vi "Configure Timebase.vi"(7 "Record Length (10000)":u32=10000 caption="Record Length (10000s)", 8 "error in (no error)":errorcluster, 9 "Position (0.0 s)":dbl=50.0, 10 "Timebase (4 ns)":dbl=4.0, 11 "VISA resource name":refnum<visa-resource-name>) -> (0 "error out":errorcluster, 3 "VISA resource name out":refnum<visa-resource-name>)   [LabVIEW 2015, in "Tektronix 7000 Series.lvlib"]
doc: "Configures the timebase and horizontal properties of an oscilloscope."
uses:
  <instrlib>/Tektronix 7000 Series/Tektronix 7000 Series.lvlib
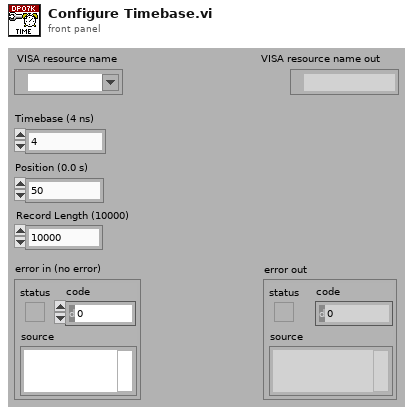
[diagram p1: front panel]
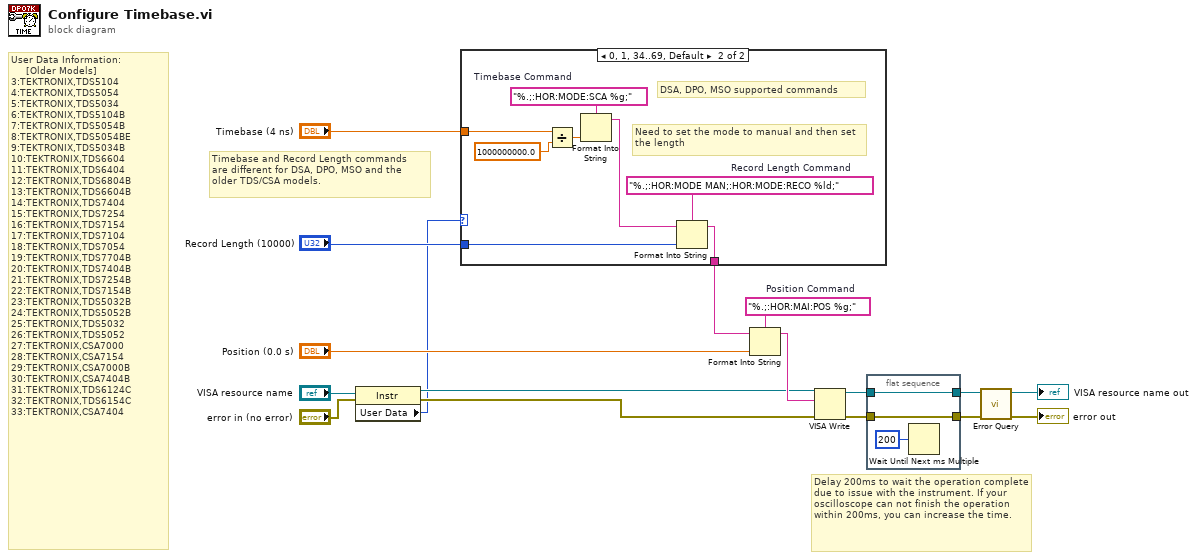
[diagram p0: block diagram]
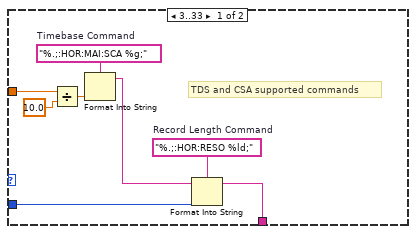
[diagram p2: hidden frame]
diagram:
  w17 = "%.;:HOR:MAI:POS %g;"  # Position Command
  # "Timebase and Record Length commands\nare different for DSA, DPO, MSO and the \nolder TDS/CSA models."
  # "User Data Information:\n     [Older Models]\n3:TEKTRONIX,TDS5104\n4:TEKTRONIX,TDS5054\n5:TEKTRONIX,TDS5034\n6:TEKTRONIX,TDS5104B\n7:TEKTRONIX,TDS5054B\n8:TEKTRONIX,TDS5054BE\n9:TEKTRONIX,TDS5034B\n10:TEKTRONIX,TDS6604\n11:TEKTRONIX,TDS6404\n12:TEKTRONIX,TDS6804B\n13:TEKTRONIX,TDS6604B\n14:TEKTRONIX,TDS7404\n15:TEKTRONIX,TDS7254\n16:TEKTRONIX,TDS7154\n17:TEKTRONIX,TDS7104\n18:TEKTRONIX,TDS7054\n19:TEKTRONIX,TDS7704B\n20:TEKTRONIX,TDS7404B\n21:TEKTRONIX,TDS7254B\n22:TEKTRONIX,TDS7154B\n23:TEKTRONIX,TDS5032B\n24:TEKTRONIX,TDS5052B\n25:TEKTRONIX,TDS5032\n26:TEKTRONIX,TDS5052\n27:TEKTRONIX,CSA7000\n28:TEKTRONIX,CSA7154\n29:TEKTRONIX,CSA7000B\n30:TEKTRONIX,CSA7404B\n31:TEKTRONIX,TDS6124C\n32:TEKTRONIX,TDS6154C\n33:TEKTRONIX,CSA7404"
  # "Delay 200ms to wait the operation complete due to issue with the instrument. If your oscilloscope can not finish the operation within 200ms, you can increase the time."
  n1 = property class="Instr"(reference="VISA resource name", error in="error in (no error)") -> (reference out=w3:refnum<visa-resource-name>, error out=w2:errorcluster, "User Data"=w1:u32)
  n2 = case shown="0, 1, 34..69, Default" w1 {
    tunnel: "Timebase (4 ns)" -> [w20 w31]
    tunnel: "Record Length (10000)" -> [w19 w28]
    tunnel: [w18 w26] -> w6
    frame 3..33 {
      w24 = "%.;:HOR:RESO %ld;"  # Record Length Command
      w25 = "%.;:HOR:MAI:SCA %g;"  # Timebase Command
      # "TDS and CSA supported commands"
      n3 = Divide(x=w20, y=10.0) -> (x/y=w22:dbl)
      n4 = Format Into String(format string=w25, w22) -> (resulting string=w21:string)  [unwired: 2 in, 1 out]
      n5 = Format Into String(format string=w24, initial string=w21, w19) -> (resulting string=w18:string)  [unwired: 1 in, 1 out]
    }
    frame 0, 1, 34..69, Default {
      w32 = "%.;:HOR:MODE MAN;:HOR:MODE:RECO %ld;"  # Record Length Command
      w33 = "%.;:HOR:MODE:SCA %g;"  # Timebase Command
      # "DSA, DPO, MSO supported commands"
      # "Need to set the mode to manual and then set the length"
      n6 = Divide(x=w31, y=1000000000.0) -> (x/y=w29:dbl)
      n7 = Format Into String(format string=w33, w29) -> (resulting string=w27:string)  [unwired: 2 in, 1 out]
      n8 = Format Into String(format string=w32, initial string=w27, w28) -> (resulting string=w26:string)  [unwired: 1 in, 1 out]
    }
  }
  n9 = Format Into String(format string=w17, initial string=w6, "Position (0.0 s)") -> (resulting string=w7:string)  [unwired: 1 in, 1 out]
  n10 = VISA Write(VISA resource name=w3, write buffer=w7, error in (no error)=w2) -> (VISA resource name out=w13:refnum<visa-resource-name>, error out=w12:errorcluster)  [unwired: 1 out]
  n11 = flat-sequence {
    tunnel: w13 -> [w35]
    tunnel: [w35] -> w10
    tunnel: w12 -> [w34]
    tunnel: [w34] -> w11
    frame #0 {
      n12 = Wait Until Next ms Multiple(millisecond multiple=u32 200) -> ()  [unwired: 1 out]
    }
  }
  n13 = call <instrlib>:"Error Query.vi"("error in (no error)"=w11, "VISA resource name"=w10) -> ("error out"=→"error out":errorcluster, "VISA resource name out"=→"VISA resource name out":refnum<visa-resource-name>)  [unwired: 6 in, 2 out]
